vi "PIDParameters.vi"(8 "error in":errorcluster, 9 "fbParams":T2, 10 "GainScale":dbl=-6.0 format="%#_13g", 11 "FPGA VI Reference In":T1) -> (0 "error out":errorcluster, 3 "FPGA VI Reference Out":T1)   [LabVIEW 2016]
uses:
  controls/FPGAVIreferenceTypeDef.ctl
  <vilib>/rvi/errors/niLvFpgaAdjustHostInterfaceError.vi
  <vilib>/Utility/error.llb/Error Cluster From Error Code.vi
  <vilib>/rvi/interface/nirviReadWriteControl/nirviReadWriteControl.xnode
  FPGA Bitfiles/qnmController797_usbRIO_controllerFPGAmu.lvbitx
  NiFpgaLv.dll
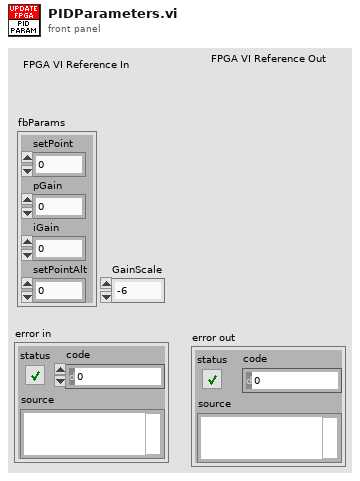
[diagram p1: front panel]
types:
  T1 = typedef "FPGAVIreferenceTypeDef.ctl" = refnum<k20>
  T2 = cluster{"setPoint":fxp<+/-,17,1>, "pGain":dbl, "iGain":dbl, "setPointAlt":fxp<+/-,17,1>}
  T3 = cluster{"setPoint":fxp<+/-,17,1>, "pGain":fxp<+/-,20,4>, "iGain":fxp<+/-,20,1>, "gainScale":i8, "setPointAlt":fxp<+/-,17,1>}
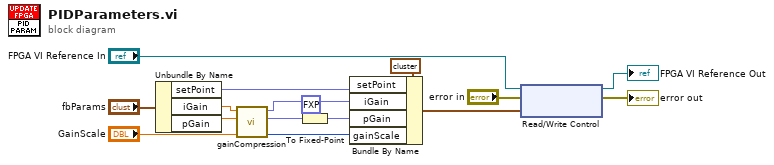
[diagram p0: block diagram]
diagram:
  n1 = Unbundle By Name("fbParams") -> ("setPoint"=w5:fxp<+/-,17,1>, "iGain"=w15:dbl, "pGain"=w16:dbl)
  n2 = call "gainCompression.vi"("compressionMin"="GainScale", "slaveInput"=w16, "masterInput"=w15) -> ("gainScale"=w12:i8, "rescaledSlave"=w13:fxp<+/-,20,1>, "rescaledMaster"=w14:fxp<+/-,20,1>)  [unwired: 6 in]
  n3 = To Fixed-Point(fixed-point type=fxp<+/-,20,4> 0.0 ("pGain"), number=w13) -> (fixed-point=w1:fxp<+/-,20,4>)
  n4 = Bundle By Name(cluster=T3 {"setPoint"=0.0, "pGain"=0.0, "iGain"=0.0, "gainScale"=0, "setPointAlt"=0.0} ("fb.p.params"), "setPoint"=w5, "iGain"=w14, "pGain"=w1, "gainScale"=w12) -> (w3:T3)
  n5 = xnode "Read/Write Control"("FPGA VI Reference In"="FPGA VI Reference In", "error in"="error in", "fb.p.params"=w3) -> ("FPGA VI Reference Out"=→"FPGA VI Reference Out":T1, "error out"=→"error out":errorcluster)
